vi "Klinger GetStatus.vi"(0 "addresse":string, 1 "error in":errorcluster) -> (2 "Message D'erreur":string, 3 "Statut":bool, 4 "Message Cont":string caption="Message de statut", 5 "error out":errorcluster)   [LabVIEW 2010]
doc: "Ce VI effectue une lecture du message de statut du contrôlleur. Celui-ci indique entre autres, si les axes sont en mouvement, la positions de chaque axe, et l'état des interrupteurs de fin de course. De plus, si une erreur c'est produite (ex: commande invalide), il retourrne un code d'erreur avec une brève description. Dans ce dernier cas, le VI rapporte le message d'erreur au VI \"Klinger ErrorHandler\"."
uses:
  <vilib>/Utility/error.llb/DialogType.ctl
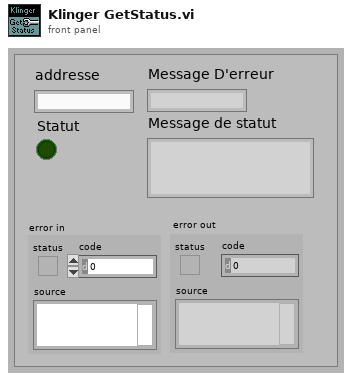
[diagram p1: front panel]
types:
  T1 = enum16{"Lit", "Fin", "Verif erreur", "fixe options", "commande ?"}
  T2 = typedef "DialogType.ctl" = u16
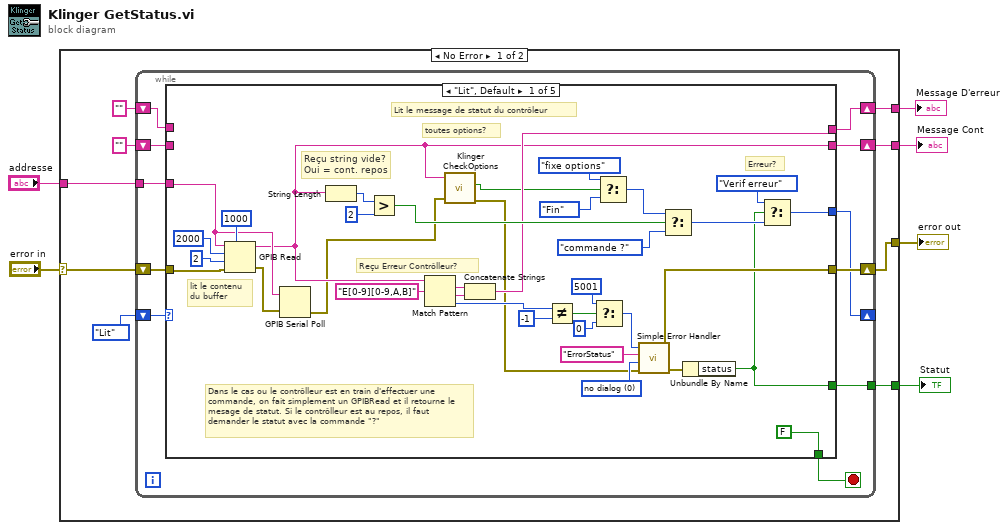
[diagram p0: block diagram]
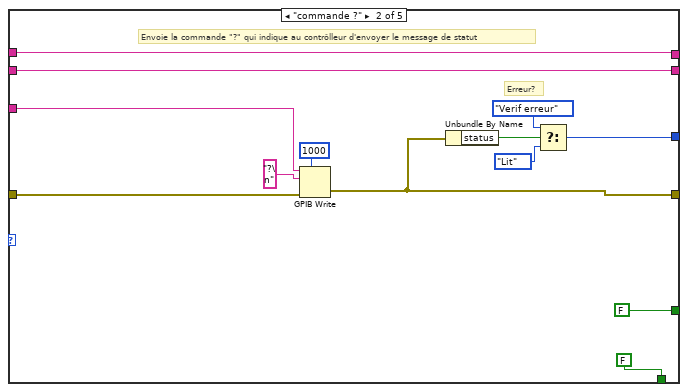
[diagram p2: hidden frame]
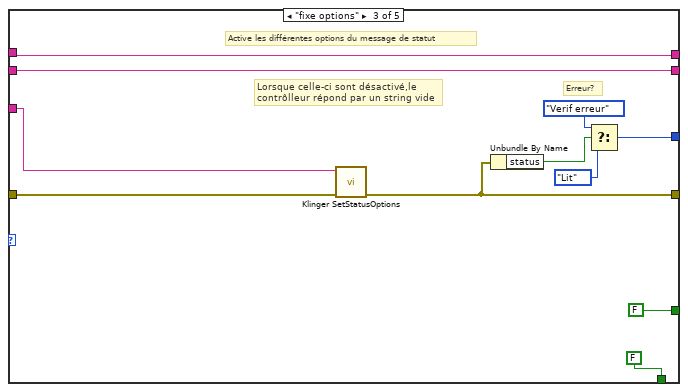
[diagram p3: hidden frame]
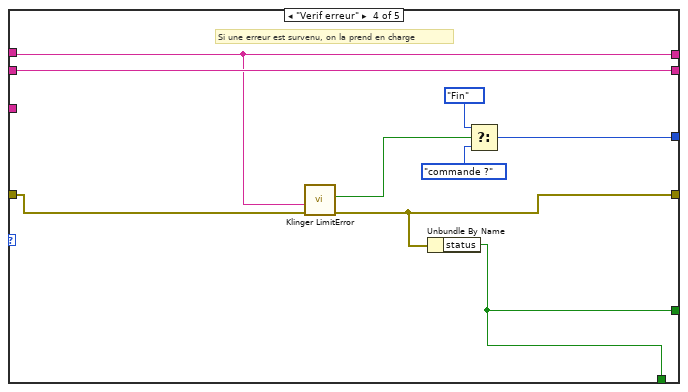
[diagram p4: hidden frame]
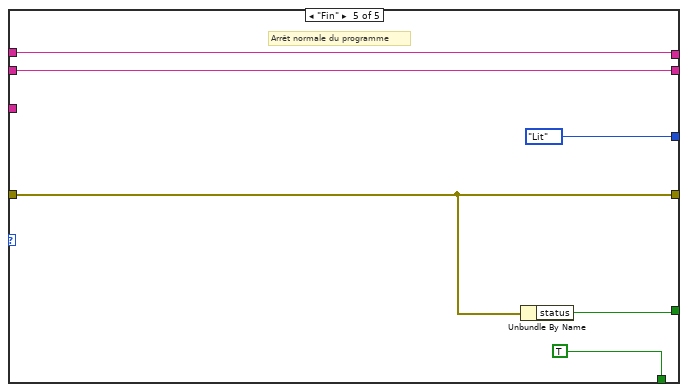
[diagram p5: hidden frame]
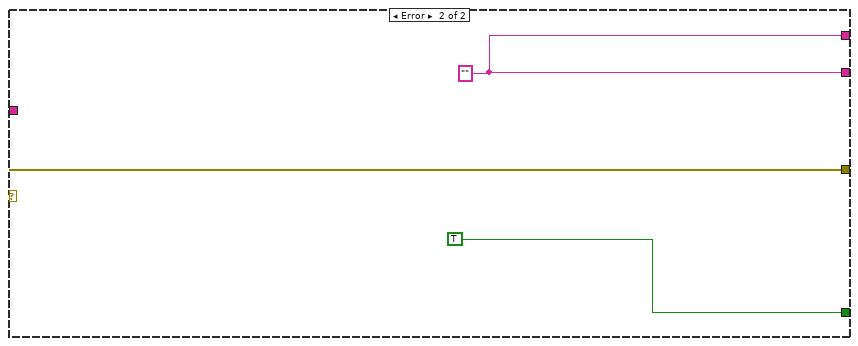
[diagram p6: hidden frame]
diagram:
  n1 = case shown="No Error" "error in" {
    selector: "error in" -> [w15 w103]
    tunnel: [w10 w101] -> w6
    tunnel: [w9 w103] -> w5
    tunnel: [w11 TRUE] -> w4
    tunnel: "addresse" -> [w13 _]
    tunnel: [w14 w101] -> w1
    frame No Error {
      n2 = while {
        tunnel: w13 -> [w25]
        tunnel: [w21] -> w11
        shift-right: [w20] -> _
        shift-left: T1."Lit" -> [w24]
        shift-right: [w23] -> w9
        shift-left: w15 -> [w26]
        shift-right: [w22] -> w14
        shift-left: "" ("data") -> [w18]
        shift-right: [w16] -> w10
        shift-left: "" -> [w17]
        stop <- w19 stop-if-true
        n3 = case shown="\"Lit\", Default" w24 {
          tunnel: w26 -> [w50 w72 w84 w94 w99]
          tunnel: [w31 w68 w82 w91 w97] -> w22
          tunnel: w25 -> [w47 w71 w85 _ _]
          tunnel: [w36 w63 w78 w87 w99] -> w23
          tunnel: [w35 FALSE FALSE ("status") w86 w100] -> w21
          tunnel: [w40 w62 w75 w93 T1."Lit"] -> w20
          tunnel: [FALSE FALSE FALSE w86 TRUE] -> w19
          tunnel: w18 -> [_ w68 w82 w91 w97]
          tunnel: w17 -> [_ w67 w83 w90 w96]
          tunnel: [w41 w67 w83 w90 w96] -> w16
          frame "Lit", Default {
            w54 = T2 0 items=["no dialog", "OK message", "continue or stop message", "OK message + warnings", "continue/stop + warnings"] ("type of dialog (OK msg:1)")
            # "toutes options?"
            # "Lit le message de statut du contrôleur"
            # "lit le contenu\ndu buffer"
            # "Dans le cas ou le contrôlleur est en train d'effectuer une commande, on fait simplement un GPIBRead et il retourne le mesage de statut. Si le contrôlleur est au repos, il faut demander le statut avec la commande \"?\""
            # "Erreur?"
            # "Reçu string vide?\nOui = cont. repos"
            # "Reçu Erreur Contrôlleur?"
            n4 = GPIB Read(0:w47, 1:2000 ("byte count"), 2:i16 2 ("mode (0)"), 3:w50, 4:1000 ("timeout ms (488.2 global)")) -> (5:w31:string, 7:w38:errorcluster)  [unwired: 1 out]
            n5 = GPIB Serial Poll(0:w47, 1:w38) -> (4:w29:errorcluster)  [unwired: 2 out]
            n6 = String Length(string=w31) -> (length=w45:i32)
            n7 = Greater?(x=w45, y=2) -> (0:w43:bool)
            n8 = Match Pattern(string=w31, regular expression="E[0-9][0-9,A,B]") -> (match substring=w59:string, after substring=w58:string, offset past match=w60:i32)  [unwired: 1 in, 1 out]
            n9 = call <userlib>:"Klinger CheckOptions.vi"("Message Cont"=w31, "error in"=w29) -> ("Statut"=w30:bool, "error out"=w28:errorcluster)  [unwired: 7 in]
            n10 = Concatenate Strings(w59, w58) -> (w41:string)
            n11 = Not Equal?(x=w60, y=-1) -> (x != y?=w53:bool)
            n12 = Select(t=5001 ("error code (no error:0)"), s=w53, f=0) -> (s? t:f=w55:i32)
            n13 = Select(t=T1."fixe options", s=w30, f=T1."Fin") -> (s? t:f=w34:T1)
            n14 = call <vilib>:"Simple Error Handler.vi"("error code (no error:0)"=w55, "error source (\" \")"="ErrorStatus" ("error source (\" \")"), "type of dialog (OK msg:1)"=w54, "error in (no error)"=w28) -> ("error out"=w36:errorcluster)  [unwired: 1 in, 4 out]
            n15 = Select(t=w34, s=w43, f=T1."commande ?") -> (s? t:f=w39:T1)
            n16 = Unbundle By Name(w36) -> ("status"=w35:bool)
            n17 = Select(t=T1."Verif erreur", s=w35, f=w39) -> (s? t:f=w40:T1)
          }
          frame "commande ?" {
            # "Erreur?"
            # "Envoie la commande \"?\" qui indique au contrôlleur d'envoyer le message de statut"
            n18 = GPIB Write(0:w71, 1:"?\n" ("data"), 3:w72, 4:1000 ("timeout ms (488.2 global)")) -> (6:w63:errorcluster)  [unwired: 1 in, 1 out]
            n19 = Unbundle By Name(w63) -> ("status"=w66:bool)
            n20 = Select(t=T1."Verif erreur", s=w66, f=T1."Lit") -> (s? t:f=w62:T1)
          }
          frame "fixe options" {
            # "Erreur?"
            # "Lorsque celle-ci sont désactivé,le contrôlleur répond par un string vide"
            # "Active les différentes options du message de statut"
            n21 = call <userlib>:"Klinger SetStatusOptions.vi"("error in"=w84, "addresse"=w85) -> ("error out"=w78:errorcluster)  [unwired: 5 in]
            n22 = Unbundle By Name(w78) -> ("status"=w79:bool)
            n23 = Select(t=T1."Verif erreur", s=w79, f=T1."Lit") -> (s? t:f=w75:T1)
          }
          frame "Verif erreur" {
            # "Si une erreur est survenu, on la prend en charge"
            n24 = call <userlib>:"Klinger LimitError.vi"("Message d'erreur"=w90, "Error In"=w94) -> ("Statut"=w92:bool, "Error out"=w87:errorcluster)  [unwired: 5 in]
            n25 = Unbundle By Name(w87) -> ("status"=w86:bool)
            n26 = Select(t=T1."Fin", s=w92, f=T1."commande ?") -> (s? t:f=w93:T1)
          }
          frame "Fin" {
            # "Arrêt normale du programme"
            n27 = Unbundle By Name(w99) -> ("status"=w100:bool)
          }
        }
      }
    }
    frame Error {
      w101 = "" ("data")
    }
  }
  "error out" <- w5
  "Statut" <- w4
  "Message D'erreur" <- w6
  "Message Cont" <- w1
